vi "Do Request.vi"(7 "Processing In":refnum<class "Processing.lvclass">, 11 "PublishConfigController in":refnum<class "PublishConfigController.lvclass">) -> (0 "error out":errorcluster, 5 "Processing":refnum<class "Processing.lvclass">)   [LabVIEW 2020, in "Vecto.lvlib" / "PublishConfigController.lvclass"]
uses:
  PublishConfigController.lvclass
  lv-http-server/HTTP Server/Processing/Processing.lvclass
  ChannelService/ChannelService.lvclass
  C:/dev/lv20CE/relink/lv-http-server/HTTP Server/Service/Service.lvclass
  Publish Config Response.ctl
  Publish Config Response Group.ctl
  Publish Config.ctl
  Group Data Type.ctl
  lv-http-server/HTTP Server/Processing/Processing.lvclass/Processing.ctl
  RemoteDataService/RemoteDataService.lvclass
  Group/Group.lvclass/Group.ctl
  Group Config/Group Config.lvclass/Group Config.ctl
  e204d32a-7846-4d24-9048-3992e314f26d.vi
  <vilib>/JDP Science/JSONtext/Variant to JSON Text.vi
  <vilib>/JDP Science/JSONtext/LVClass Serializer/JSONtext LVClass Serializer.lvclass
  PublishConfigController.lvclass/PublishConfigController.ctl
  Group Config/Group Config.lvclass
  Channel Config/Channel Config.lvclass
  VectoConfig/VectoConfig.lvlib
  Vecto.lvlib
  lv-http-util/HTTP Utils/Response/Response.lvclass
  Group/Group.lvclass
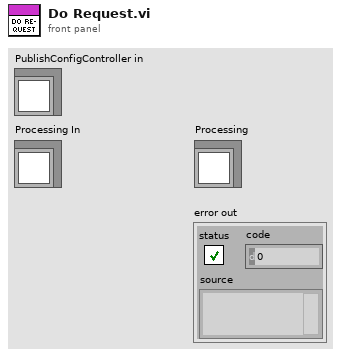
[diagram p1: front panel]
types:
  T1 = typedef "Vecto.lvlib/Publish Config Response.ctl" = cluster{"Groups":T2[]}
  T2 = typedef "Vecto.lvlib/Publish Config Response Group.ctl" = cluster{"Name":string, "Endpoint":T3, "OwningTask":string, "Data Type":T4, "Channels":cluster{"Name":string, "Resource":string}[]}
  T3 = typedef "VectoConfig.lvlib/Publish Config.ctl" = cluster{"Address":string, "Port":u16}
  T4 = typedef "VectoConfig.lvlib/Group Data Type.ctl" = enum16{"Double", "String", "Bool"}
  T5 = typedef "VectoConfig.lvlib/Channel Info.ctl" = cluster{"Name":string, "Group":string, "Owning Node":string, "Owning Task":string, "Resource":string}
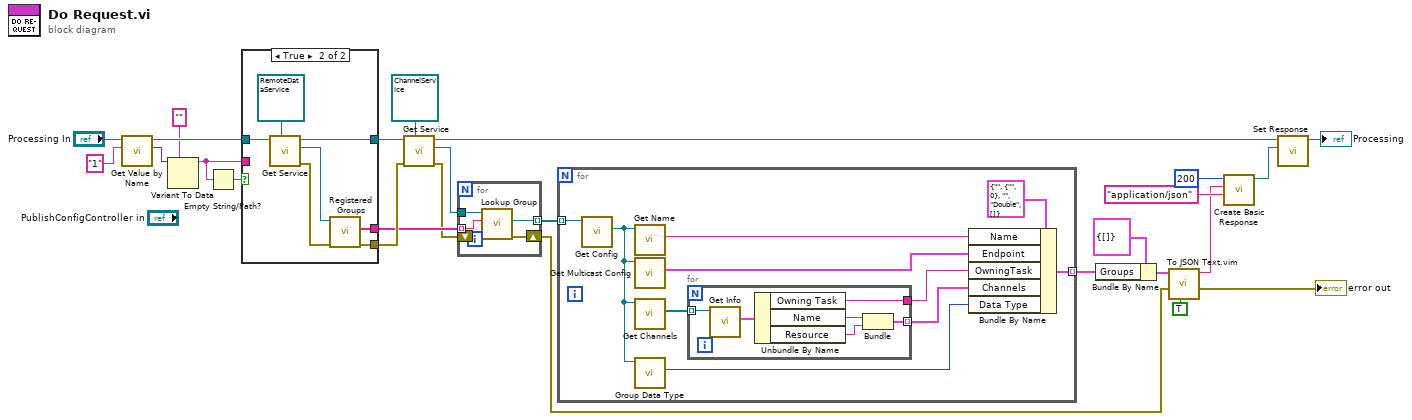
[diagram p0: block diagram]
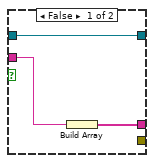
[diagram p2: hidden frame]
diagram:
  n1 = call "Get Value by Name.vi"("Name"="1", "Processing in"="Processing In") -> ("Value"=w9:variant, "Processing out"=w10:refnum<class "Processing.lvclass">)  [unwired: 7 in, 1 out]
  n2 = Variant To Data(type="", Variant=w9) -> (data=w7:string)  [unwired: 1 in, 1 out]
  n3 = Empty String/Path?(string/path=w7) -> (empty?=w6:bool)
  n4 = case shown="True" w6 {
    tunnel: [_ w36] -> w26
    tunnel: [w27 w33] -> w25
    tunnel: [w28 w32] -> w23
    tunnel: w10 -> [w27 w30]
    tunnel: w7 -> [w29 _]
    frame False {
      n5 = Build Array(w29) -> (w28:string[])
    }
    frame True {
      n6 = call "Get Service.vi"("Service Type"=refnum<class "RemoteDataService.lvclass"> refnum ("Vecto.lvlib:RemoteDataService.lvclass"), "Processing in"=w30) -> ("error out"=w31:errorcluster, "Service"=w34:refnum<class "RemoteDataService.lvclass">, "Processing out"=w33:refnum<class "Processing.lvclass">)  [unwired: 7 in]
      n7 = call "Registered Groups.vi"("error in (no error)"=w31, "RemoteDataService in"=w34) -> ("error out"=w36:errorcluster, "Registered Groups"=w32:string[])  [unwired: 7 in, 1 out]
    }
  }
  n8 = call "Get Service.vi"("Service Type"=refnum<class "ChannelService.lvclass"> refnum ("Vecto.lvlib:ChannelService.lvclass"), "error in (no error)"=w26, "Processing in"=w25) -> ("error out"=w13:errorcluster, "Service"=w22:refnum<class "ChannelService.lvclass">, "Processing out"=w15:refnum<class "Processing.lvclass">)  [unwired: 6 in]
  n9 = for {
    tunnel: w23 -> [w41] mode=indexing
    tunnel: w22 -> [w40]
    tunnel: [w39] -> w21 mode=indexing
    shift-right: [w37] -> w4
    shift-left: w13 -> [w38]
    n10 = call "Lookup Group.vi"("error in (no error)"=w38, "Group Name"=w41, "ChannelService in"=w40) -> ("error out"=w37:errorcluster, "Group"=w39:refnum<class "Group.lvclass">)  [unwired: 6 in, 1 out]
  }
  n11 = for {
    tunnel: w21 -> [w51] mode=indexing
    tunnel: [w46] -> w19 mode=indexing
    n12 = call "Get Config.vi"("Group in"=w51) -> ("Config"=w45:refnum<class "Group Config.lvclass">)  [unwired: 8 in, 2 out]
    n13 = call "Get Name.vi"("Group Config in"=w45) -> ("Name"=w48:string)  [unwired: 8 in, 2 out]
    n14 = call "Get Multicast Config.vi"("Group Config in"=w45) -> ("Multicast Config"=w47:T3)  [unwired: 8 in, 2 out]
    n15 = call "Get Channels.vi"("Group Config in"=w45) -> ("Channels"=w50:refnum<class "Channel Config.lvclass">[])  [unwired: 8 in, 2 out]
    n16 = call "Group Data Type.vi"("Group Config in"=w45) -> ("Data Type"=w44:T4)  [unwired: 8 in, 2 out]
    n17 = for {
      tunnel: w50 -> [w57] mode=indexing
      tunnel: [w55] -> w43
      tunnel: [w52] -> w42 mode=indexing
      n18 = call "Get Info.vi"("Channel Config in"=w57) -> ("Info"=w56:T5)  [unwired: 8 in, 2 out]
      n19 = Unbundle By Name(w56) -> ("Owning Task"=w55:string, "Name"=w54:string, "Resource"=w53:string)
      n20 = Bundle("Name"=w54, "Resource"=w53) -> (w52:cluster{"Name":string, "Resource":string})  [unwired: 1 in]
    }
    n21 = Bundle By Name(cluster=T2 {"Name"="", "Endpoint"={"Address"="", "Port"=0}, "OwningTask"="", "Data Type"=enum."Double", "Channels"=[]} ("Publish Config Group"), "Name"=w48, "Endpoint"=w47, "OwningTask"=w43, "Channels"=w42, "Data Type"=w44) -> (w46:T2)
  }
  n22 = Bundle By Name(cluster=T1 {"Groups"=[]} ("Publish Config Response"), "Groups"=w19) -> (w5:T1)
  n23 = call "To JSON Text.vim"("Pretty Print?"=TRUE, "error in (no error)"=w4, "Anything"=w5) -> ("error out"=→"error out":errorcluster, "<JSON>"=w3:string)  [unwired: 7 in]
  n24 = call "Create Basic Response.vi"("Content-Type (text/plain)"="application/json", "Payload"=w3, "Status Code"=u16 200) -> ("Response out"=w16:refnum<class "Response.lvclass">)  [unwired: 7 in, 1 out]
  n25 = call "Set Response.vi"("Response"=w16, "Processing in"=w15) -> ("Processing out"=→"Processing":refnum<class "Processing.lvclass">)  [unwired: 9 in]
